vi "read config.vi"(8 "error in (no error)":errorcluster, 10 "config file path":path, 11 "USB IO in":refnum<class "USB IO.lvclass">) -> (0 "error out":errorcluster, 3 "USB IO out":refnum<class "USB IO.lvclass">)   [LabVIEW 2025, in "USB IO.lvclass"]
uses:
  USB IO.lvclass
  USB IO.lvclass/USB IO.ctl
  9b8b088c-8bc7-4bef-a6f3-163340907b3e.vi
  <vilib>/JDP Science/JSONtext/JSON text to Variant.vi
  <vilib>/JDP Science/JSONtext/LVClass Serializer/JSONtext LVClass Serializer.lvclass
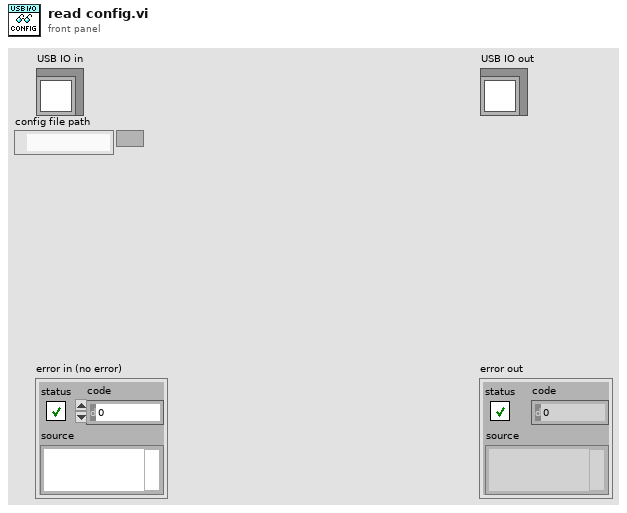
[diagram p1: front panel]
types:
  T1 = cluster{"Device_Name":string, "Inputs_Name":string}
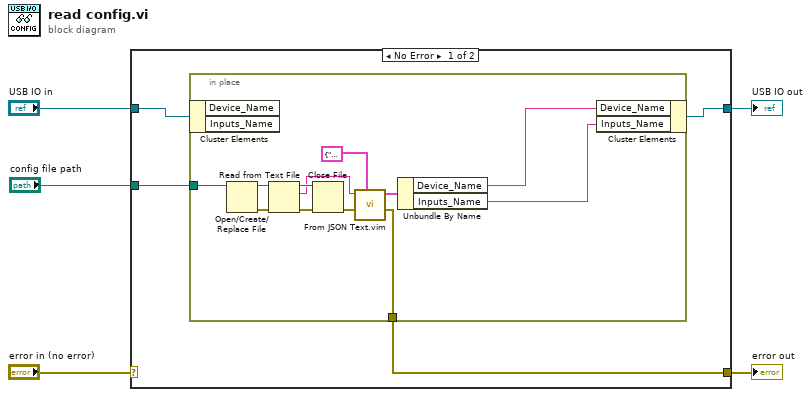
[diagram p0: block diagram]
diagram:
  n1 = case shown="No Error" "error in (no error)" {
    selector: "error in (no error)" -> [_ w23]
    tunnel: [w6 w23] -> w4
    tunnel: [w8 w22] -> w2
    tunnel: "USB IO in" -> [w9 w22]
    tunnel: "config file path" -> [w7 _]
    frame No Error {
      n2 = in-place {
        in-place-border: w7 -> [w15]
        in-place-border: [w11] -> w6
        n3 = in-place-cluster #1(w9) -> ()  [unwired: 2 out]
        n4 = Open/Create/Replace File(file path (use dialog)=w15) -> (refnum out=w18:refnum<file>, error out=w21:errorcluster)  [unwired: 5 in, 1 out]
        n5 = Read from Text File(file (use dialog)=w18, error in=w21) -> (refnum out=w19:refnum<file>, text=w17:string, error out=w20:errorcluster)  [unwired: 2 in, 1 out]
        n6 = Close File(refnum=w19, error in=w20) -> (error out=w16:errorcluster)  [unwired: 1 out]
        n7 = call "From JSON Text.vim"("Data Type and Default Value"=T1 {"Device_Name"="", "Inputs_Name"=""}, "error in (no error)"=w16, "JSON"=w17) -> ("error out"=w11:errorcluster, "Data out"=w14:T1)  [unwired: 7 in]
        n8 = Unbundle By Name(w14) -> ("Device_Name"=w12:string, "Inputs_Name"=w10:string)
        n9 = in-place-cluster #1("Device_Name"=w12, "Inputs_Name"=w10) -> (w8:refnum<class "USB IO.lvclass">)
      }
    }
    frame Error {
    }
  }
  "error out" <- w4
  "USB IO out" <- w2
